vi "ConnectCameraRslt.vi"(8 "error in (no error)":errorcluster, 11 "CameraTestingUI in":refnum<class "CameraTestingUI.lvclass">) -> (0 "error out":errorcluster, 3 "CameraTestingUI out":refnum<class "CameraTestingUI.lvclass">)   [LabVIEW 2020, in "CameraTestingUI.lvlib" / "CameraTestingUI.lvclass"]
uses:
  CameraTestingUI.lvclass
  CameraTestingUI.lvclass/CameraTestingUI.ctl
  Private/TypeDef/ConnectionStatus.ctl
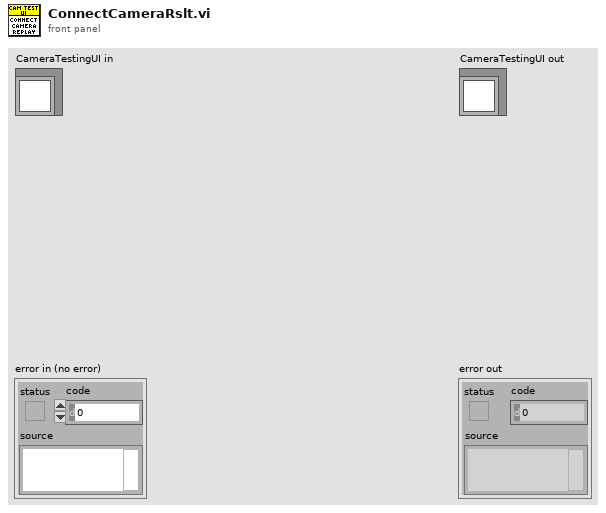
[diagram p1: front panel]
types:
  T1 = enum8{"Enabled", "Disabled", "Disabled and Grayed Out"}
  T2 = typedef "CameraTestingUI.lvlib/CameraTestingUI.lvclass/ConnectionStatus.ctl" = u16
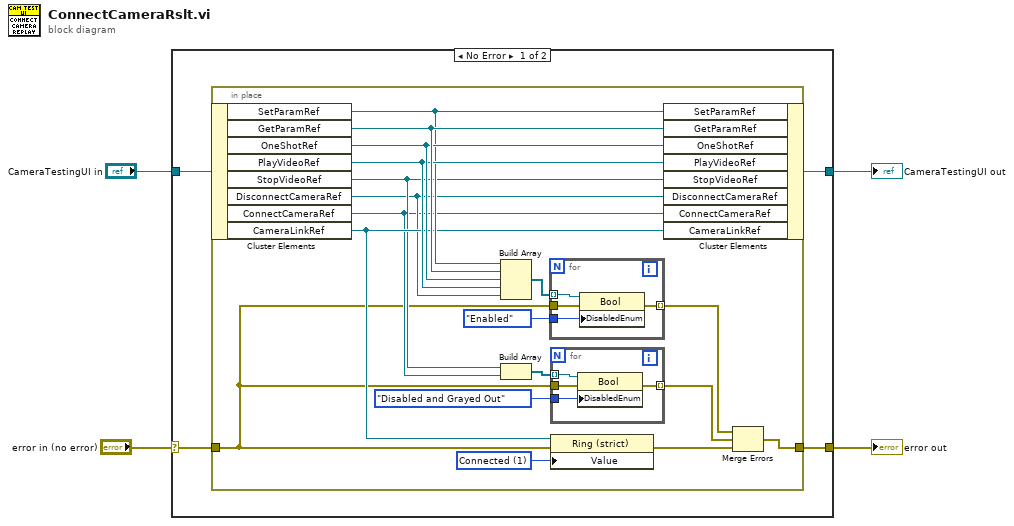
[diagram p0: block diagram]
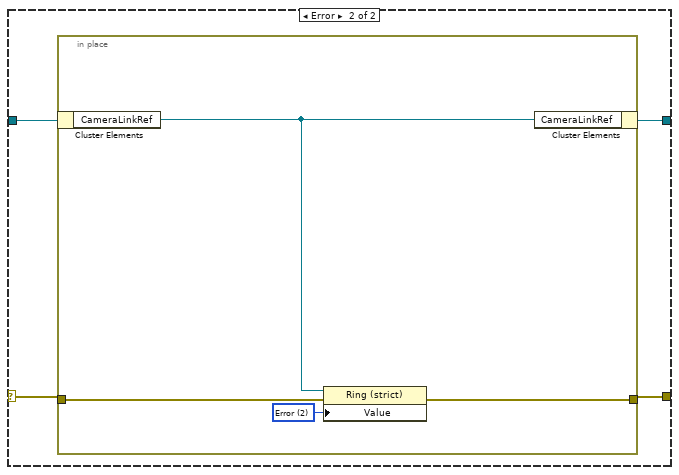
[diagram p2: hidden frame]
diagram:
  n1 = case shown="No Error" "error in (no error)" {
    selector: "error in (no error)" -> [w6 w37]
    tunnel: "CameraTestingUI in" -> [w8 w38]
    tunnel: [w7 w35] -> w2
    tunnel: [w5 w36] -> w1
    frame No Error {
      n2 = in-place {
        in-place-border: w6 -> [w12]
        in-place-border: [w19] -> w5
        w17 = T2 1 items=["Disconnected", "Connected", "Error", "", ""] ("Value")
        n3 = in-place-cluster #1(w8) -> ("SetParamRef"=w23:refnum<vi>, "GetParamRef"=w26:refnum<vi>, "OneShotRef"=w25:refnum<vi>, "PlayVideoRef"=w24:refnum<vi>, "StopVideoRef"=w15:refnum<vi>, "DisconnectCameraRef"=w14:refnum<vi>, "ConnectCameraRef"=w13:refnum<vi>, "CameraLinkRef"=w18:refnum<vi>)
        n4 = Build Array(w23, w26, w25, w24, w14) -> (w22:refnum<vi>[])
        n5 = Build Array(w15, w13) -> (w16:refnum<vi>[])
        n6 = for {
          tunnel: w22 -> [w34] mode=indexing
          tunnel: w12 -> [w33]
          tunnel: [w32] -> w21 mode=indexing
          tunnel: T1."Enabled" ("Disabled") -> [w31]
          n7 = property class="Bool"(reference=w34, error in=w33, "DisabledEnum"=w31) -> (error out=w32:errorcluster)  [unwired: 1 out]
        }
        n8 = for {
          tunnel: w16 -> [w30] mode=indexing
          tunnel: w12 -> [w29]
          tunnel: [w28] -> w9 mode=indexing
          tunnel: T1."Disabled and Grayed Out" ("Disabled") -> [w27]
          n9 = property class="Bool"(reference=w30, error in=w29, "DisabledEnum"=w27) -> (error out=w28:errorcluster)  [unwired: 1 out]
        }
        n10 = property class="Ring (strict)"(reference=w18, error in=w12, "Value"=w17) -> (error out=w20:errorcluster)  [unwired: 1 out]
        n11 = in-place-cluster #1("SetParamRef"=w23, "GetParamRef"=w26, "OneShotRef"=w25, "PlayVideoRef"=w24, "StopVideoRef"=w15, "DisconnectCameraRef"=w14, "ConnectCameraRef"=w13, "CameraLinkRef"=w18) -> (w7:refnum<class "CameraTestingUI.lvclass">)
        n12 = Merge Errors(w21, w9, w20) -> (w19:errorcluster)
      }
    }
    frame Error {
      n13 = in-place {
        in-place-border: w37 -> [w41]
        in-place-border: [w40] -> w36
        w42 = T2 2 items=["Disconnected", "Connected", "Error", "", ""] ("Value")
        n14 = in-place-cluster #2(w38) -> ("CameraLinkRef"=w39:refnum<vi>)
        n15 = property class="Ring (strict)"(reference=w39, error in=w41, "Value"=w42) -> (error out=w40:errorcluster)  [unwired: 1 out]
        n16 = in-place-cluster #2("CameraLinkRef"=w39) -> (w35:refnum<class "CameraTestingUI.lvclass">)
      }
    }
  }
  "error out" <- w1
  "CameraTestingUI out" <- w2
